vi "libdaq_dac_set_value.vi"(0 "error in (no error)":errorcluster, 1 "device_name":string, 2 "module_name":string, 4 "value":dbl) -> (14 "error out":errorcluster, 15 "device_name":string, 16 "module_name":string)   [LabVIEW 2010, in "libdaqVI.lvlib"]
doc: "设置DAC模块的输出电压值，该函数适用于控制DAC输出直流电压信号或者缓变的电压信号"
uses:
  libdaqVI.lvlib
  dll/daqlib.dll
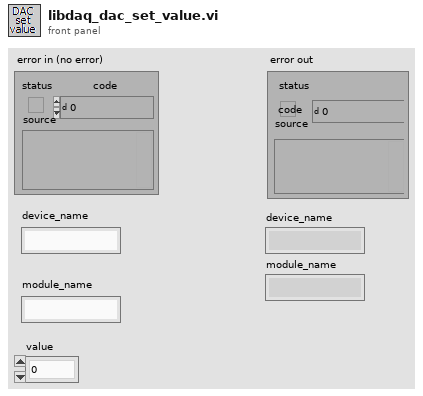
[diagram p1: front panel]
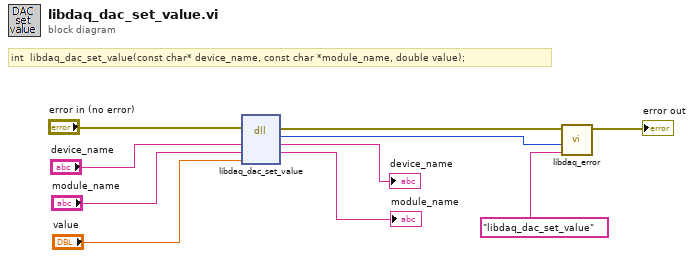
[diagram p0: block diagram]
diagram:
  # "int  libdaq_dac_set_value(const char* device_name, const char *module_name, double value);"
  n1 = dll-call lib="E:/Product/Example/DAQ-USB3212/Labview/labview_2010/libdaqVI/dll/daqlib.dll" fn="libdaq_dac_set_value"(error in="error in (no error)", "device_name"="device_name", "module_name"="module_name", "value"="value") -> (error out=w6:errorcluster, "return type"=w4:i32, "device_name"=→"device_name":string, "module_name"=→"module_name":string)  [unwired: 3 in, 1 out]
  n2 = call "libdaq_error.vi"("error source"="libdaq_dac_set_value", "error code"=w4, "错误输入（无错误）"=w6) -> ("错误输出"=→"error out":errorcluster)  [unwired: 8 in]
